vi "daqusb6251.vi"() -> ()   [LabVIEW 2021]
panel:
  out "Final time [s]":dbl
  out "Min":dbl
  out "Sec":dbl
  out "H":dbl
  out "Iteration":i32
  out "Waveform Chart 8":dynamicdata(graph)=[{"t0"=timestamp(3730382840.471822 s since 1904-01-01), "dt"=1.0, "Y"=[0.00040631009132433525]}]
  out "Waveform Chart 7":dynamicdata(graph)=[{"t0"=timestamp(3730382840.471822 s since 1904-01-01), "dt"=1.0, "Y"=[0.00040631009132433525]}]
  out "Waveform Chart 6":dynamicdata(graph)=[{"t0"=timestamp(3730382840.471822 s since 1904-01-01), "dt"=1.0, "Y"=[0.00040631009132433525]}]
  out "Waveform Chart 5":dynamicdata(graph)=[{"t0"=timestamp(3730382840.471822 s since 1904-01-01), "dt"=1.0, "Y"=[0.05613982647020779]}]
  out "Waveform Chart 4":dynamicdata(graph)=[{"t0"=timestamp(3730382840.471822 s since 1904-01-01), "dt"=1.0, "Y"=[0.07804664041667872]}]
  out "Waveform Chart 3":dynamicdata(graph)=[{"t0"=timestamp(3730382840.471822 s since 1904-01-01), "dt"=1.0, "Y"=[0.00040631009132433525]}]
  out "Waveform Chart 2":dynamicdata(graph)=[{"t0"=timestamp(3730382840.471822 s since 1904-01-01), "dt"=1.0, "Y"=[-0.00023800805463109788]}]
  in  "device name":tag="Dev1"
  in  "number of samples":i32=1
  in  "rate":dbl=100.0
  out "Waveform Chart":dynamicdata(graph)=[{"t0"=timestamp(3730382840.471822 s since 1904-01-01), "dt"=1.0, "Y"=[-0.23734714614383248]}]
  in  "Stop":bool
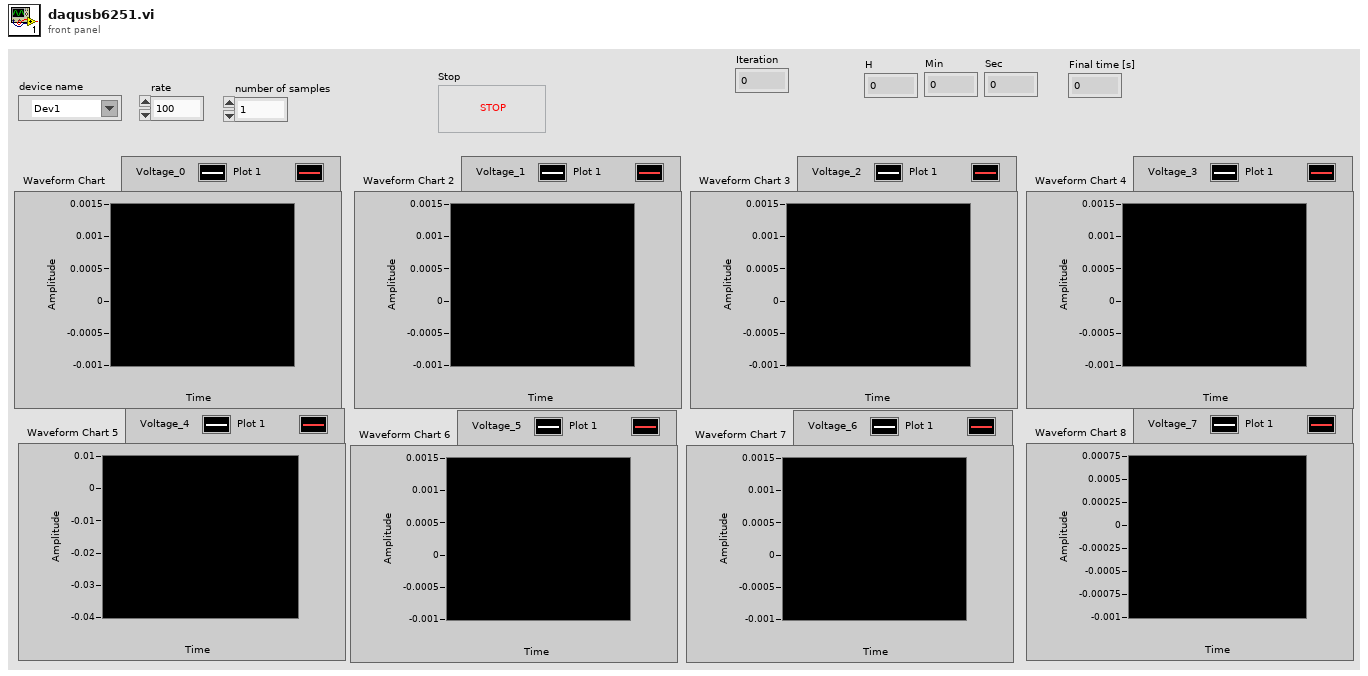
[diagram p1: front panel]
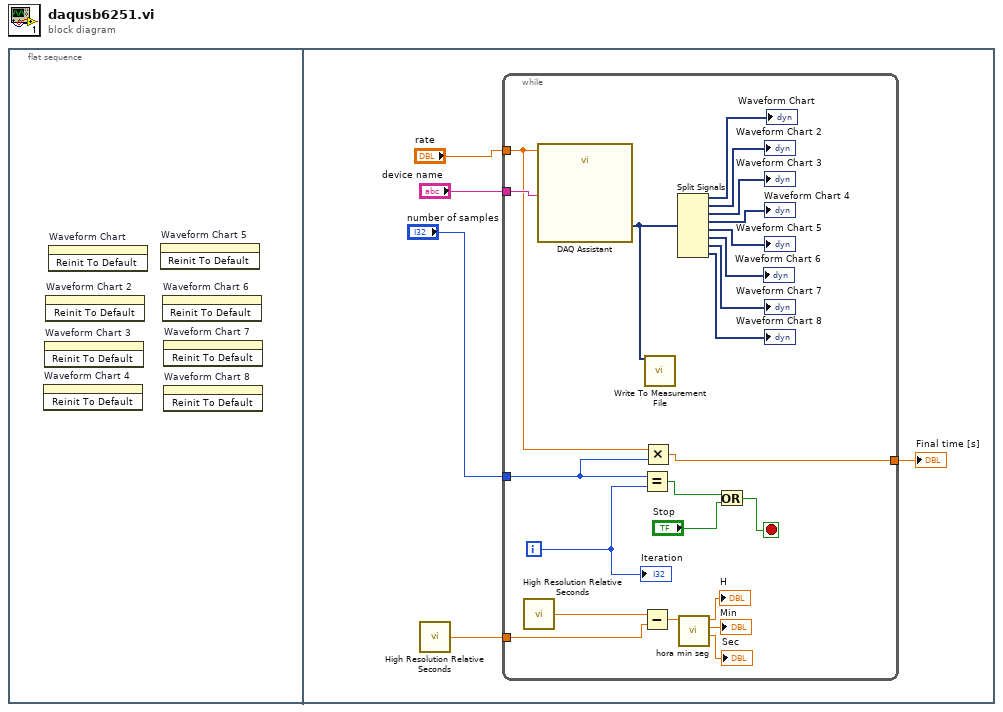
[diagram p0: block diagram]
diagram:
  n1 = flat-sequence {
    frame #0 {
      n2 = invoke on="Waveform Chart 4" class="WFChart (strict)" method="Reinit To Default"() -> ()  [unwired: 3 in, 3 out]
      n3 = invoke on="Waveform Chart 3" class="WFChart (strict)" method="Reinit To Default"() -> ()  [unwired: 3 in, 3 out]
      n4 = invoke on="Waveform Chart 2" class="WFChart (strict)" method="Reinit To Default"() -> ()  [unwired: 3 in, 3 out]
      n5 = invoke on="Waveform Chart" class="WFChart (strict)" method="Reinit To Default"() -> ()  [unwired: 3 in, 3 out]
      n6 = invoke on="Waveform Chart 5" class="WFChart (strict)" method="Reinit To Default"() -> ()  [unwired: 3 in, 3 out]
      n7 = invoke on="Waveform Chart 6" class="WFChart (strict)" method="Reinit To Default"() -> ()  [unwired: 3 in, 3 out]
      n8 = invoke on="Waveform Chart 7" class="WFChart (strict)" method="Reinit To Default"() -> ()  [unwired: 3 in, 3 out]
      n9 = invoke on="Waveform Chart 8" class="WFChart (strict)" method="Reinit To Default"() -> ()  [unwired: 3 in, 3 out]
    }
    frame #1 {
      n10 = call <vilib>:"High Resolution Relative Seconds.vi"() -> ("relative seconds"=w3:dbl)
      n11 = while {
        tunnel: "device name" -> [w27]
        tunnel: "number of samples" -> [w14]
        tunnel: [w13] -> w2
        tunnel: w3 -> [w7]
        tunnel: "rate" -> [w6]
        i -> [w16]
        stop <- w17 stop-if-true
        n12 = call <vilib>:"High Resolution Relative Seconds.vi"() -> ("relative seconds"=w12:dbl)
        n13 = call "DAQ Assistant"("rate"=w6, "device name"=w27) -> ("data"=w26:dynamicdata)  [unwired: 14 in, 3 out]
        n14 = Equal?(x=w14, y=w16) -> (x = y?=w15:bool)
        n15 = Subtract(x=w12, y=w7) -> (x-y=w11:dbl)
        n16 = Multiply(x=w6, y=w14) -> (x*y=w13:dbl)
        n17 = call "Write To Measurement File"("Signals"=w26) -> ()  [unwired: 16 in, 3 out]
        n18 = Split Signals(w26) -> (→"Waveform Chart":dynamicdata, →"Waveform Chart 2":dynamicdata, →"Waveform Chart 3":dynamicdata, →"Waveform Chart 4":dynamicdata, →"Waveform Chart 5":dynamicdata, →"Waveform Chart 6":dynamicdata, →"Waveform Chart 7":dynamicdata, →"Waveform Chart 8":dynamicdata)  [unwired: 8 in]
        n19 = call "hora min seg.vi"("Total time in seconds"=w11) -> ("Sec"=→"Sec":dbl, "Min"=→"Min":dbl, "H"=→"H":dbl)  [unwired: 8 in]
        n20 = Or(x=w15, y="Stop") -> (x .or. y?=w17:bool)
        "Iteration" <- w16
      }
      "Final time [s]" <- w2
    }
  }
